vi "Periodic Tasks.vi"(8 "error in":errorcluster) -> ()   [LabVIEW 2017]
doc: "This VI runs in parallel to other tasks. It can contain as many user-defined periodic loops as you need. These can carry out PID or other sorts of timed response."
uses:
  <vilib>/Rock Robotics/WPI/ThirdParty/Phoenix-LabVIEW/Motor Controller/Controls/CTRE_Phoenix_MotorControl_FeedbackDevice.ctl
  <vilib>/Rock Robotics/WPI/ThirdParty/Phoenix-LabVIEW/Motor Controller/Controls/CTRE_Phoenix_MotorControl_StatusFrameEnhanced.ctl
  <vilib>/Rock Robotics/WPI/ThirdParty/Phoenix-LabVIEW/Motor Controller/Controls/CTRE_Phoenix_MotorControl_ControlMode.ctl
  <vilib>/Rock Robotics/WPI/ThirdParty/Phoenix-LabVIEW/Motor Controller/Controls/CTRE_Phoenix_MotorControl_TrajectoryPointTimeDur.ctl
  <vilib>/Rock Robotics/WPI/Utilities/WPI_GetSetVariantRefNum.vi
  <vilib>/Utility/file.llb/Read Delimited Spreadsheet (DBL).vi
panel:
  out "all rows 2":dbl[][](array[numeric])
  out "all rows":dbl[][](array[numeric])
  out "Mot Prof Active Velocity 2":dbl
  out "Mot Prof Active Position 2":dbl
  out "Mot Prof  Is Under Run 2":bool
  out "Mot Prof  Has Under Run 2":bool
  out "Mot Prof Active Is Last 2":bool
  out "Mot Prof Active Is Valid 2":bool
  out "Top Mot Prof Count 2":i32
  out "Btm Mot Prof Count 2":i32
  out "Btm Mot Prof Count":i32
  out "Sensor Out Of Phase":bool
  out "Loop Time":u32
  out "Points in the CSV":i32
  out "Mot Prof Active Position":dbl
  out "Mot Prof Active Velocity":dbl
  out "Top Mot Prof Count":i32
  out "Mot Prof Active Is Valid":bool
  out "Mot Prof Active Is Last":bool
  out "Mot Prof  Has Under Run":bool
  out "Mot Prof  Is Under Run":bool
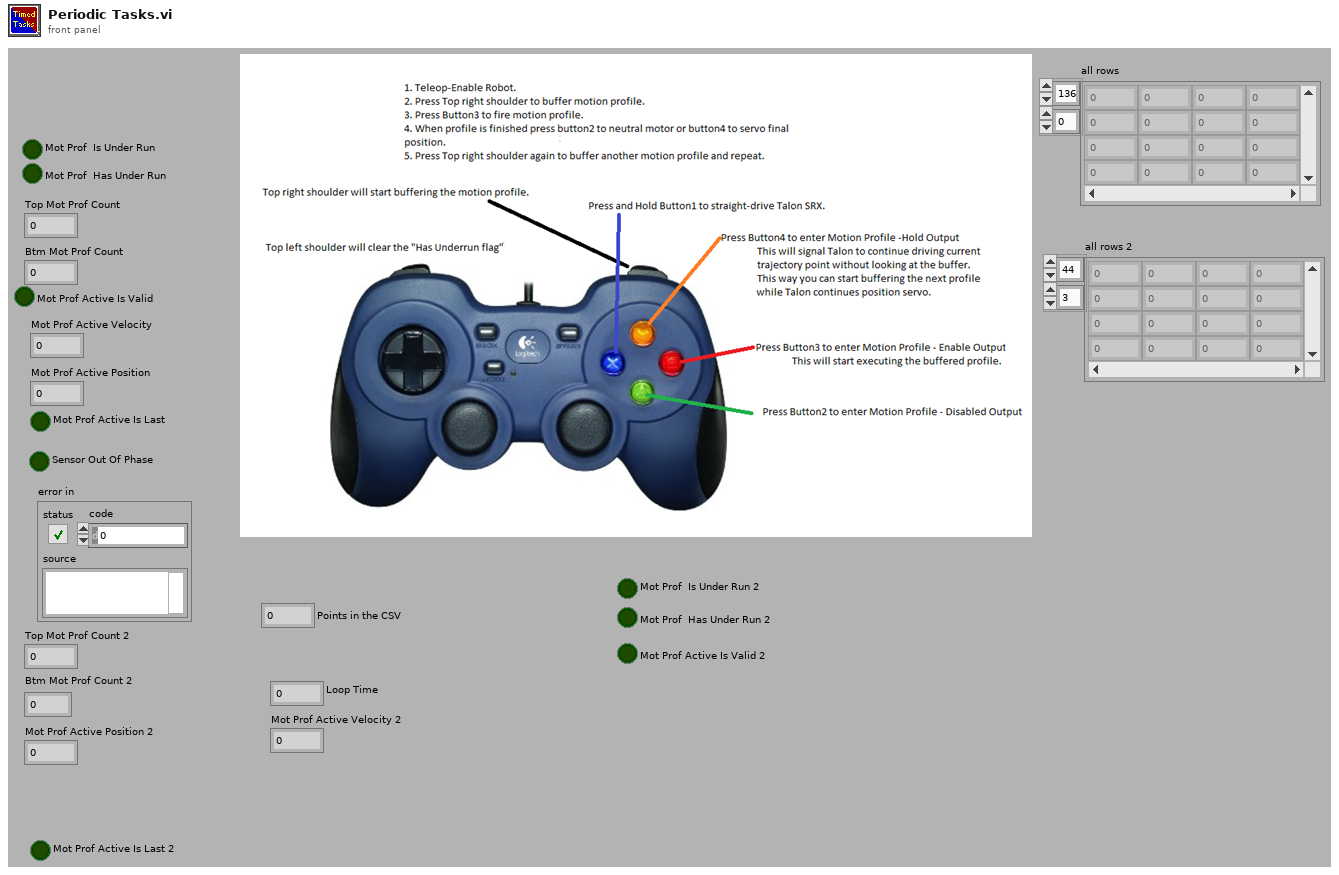
[diagram p1: front panel]
types:
  T1 = typedef "CTRE_Phoenix_MotorControl_StatusFrameEnhanced.ctl" = u16
  T2 = typedef "CTRE_Phoenix_MotorControl_FeedbackDevice.ctl" = i8
  T3 = typedef "WPI_MotorControlDeviceRef.ctl" = cluster{"DeviceStatus":errorcluster, "Type":T4, "PWM":cluster{"PWM Channel":T5, "DeadBand":T6}, "CAN":cluster{"Device Number":u8, "SetOutput VI Ref":variant, "GetOutput VI Ref":variant, "Enable VI Ref":variant, "Disable VI Ref":variant, "Data":variant}, "Invert":bool, "DIO PWM":cluster{"PWM \"Enable\" Channel":T5, "DIOChannel":T7, "PWM Rate":dbl}}
  T4 = typedef "WPI_MotorControlType.ctl" = enum16{"PWM", "CAN", "DIO PWM"}
  T5 = typedef "FPGA_DIOPWMChannel.ctl" = enum8{"PWM 0", "PWM 1", "PWM 2", "PWM 3", "PWM 4", "PWM 5", "PWM 6", "PWM 7", "PWM 8", "PWM 9", "PWM MXP 0", "PWM MXP 1", "PWM MXP 2", "PWM MXP 3", "PWM MXP 4", "PWM MXP 5", "PWM MXP 6", "PWM MXP 7", "PWM MXP 8", "PWM MXP 9", "Invalid"}
  T6 = typedef "WPI_PWMDeadband.ctl" = cluster{"Name":string, "maxPositivePwm":i32, "minPositivePwm":i32, "centerPwm":i32, "maxNegativePwm":i32, "minNegativePwm":i32, "angularRange":u16}
  T7 = typedef "FPGA_DIOChannel.ctl" = enum8{"DIO 0", "DIO 1", "DIO 2", "DIO 3", "DIO 4", "DIO 5", "DIO 6", "DIO 7", "DIO 8", "DIO 9", "DIO MXP 0", "DIO MXP 1", "DIO MXP 2", "DIO MXP 3", "DIO MXP 4", "DIO MXP 5", "DIO MXP 6", "DIO MXP 7", "DIO MXP 8", "DIO MXP 9", "DIO MXP 10", "DIO MXP 11", "DIO MXP 12", "DIO MXP 13", "DIO MXP 14", "DIO MXP 15", "SPI Port CS1", "SPI Port CS2", "SPI Port CS3", "SPI Port MISO", "SPI Port MOSI", "Invalid"}
  T8 = typedef "WPI_JoystickDevRef.ctl" = cluster{"Device":T9}
  T9 = typedef "WPI_JoystickDeviceEnum.ctl" = enum16{"USB 0", "USB 1", "USB 2", "USB 3", "USB 4", "USB 5"}
  T10 = typedef "CTRE_Phoenix_MotorControl_ControlMode.ctl" = u16
  T11 = cluster{"Under Voltage":bool, "Forward Limit Switch":bool, "Reverse Limit Switch":bool, "Forward Soft Limit":bool, "Reverse Soft Limit":bool, "Hardware Failure":bool, "Reset During Enable":bool, "Sensor Overflow":bool, "Sensor Out of Phase":bool, "Hardware ESD Reset":bool, "Remote Loss of Signal":bool}
  T12 = cluster{"Top Buffer Remaining":i32, "Top Buffer Count":i32, "Bottom Buffer Count":i32, "Has Underrun?":bool, "Is Underrun?":bool, "Active Point Valid?":bool, "Is Last?":bool, "Profile Slot Select 0":i32, "Output Enable":i32, "Time Duration (ms)":i32, "Profile Slot Select 1":i32}
  T13 = typedef "CTRE_Phoenix_MotorControl_TrajectoryPointTimeDur.ctl" = i32
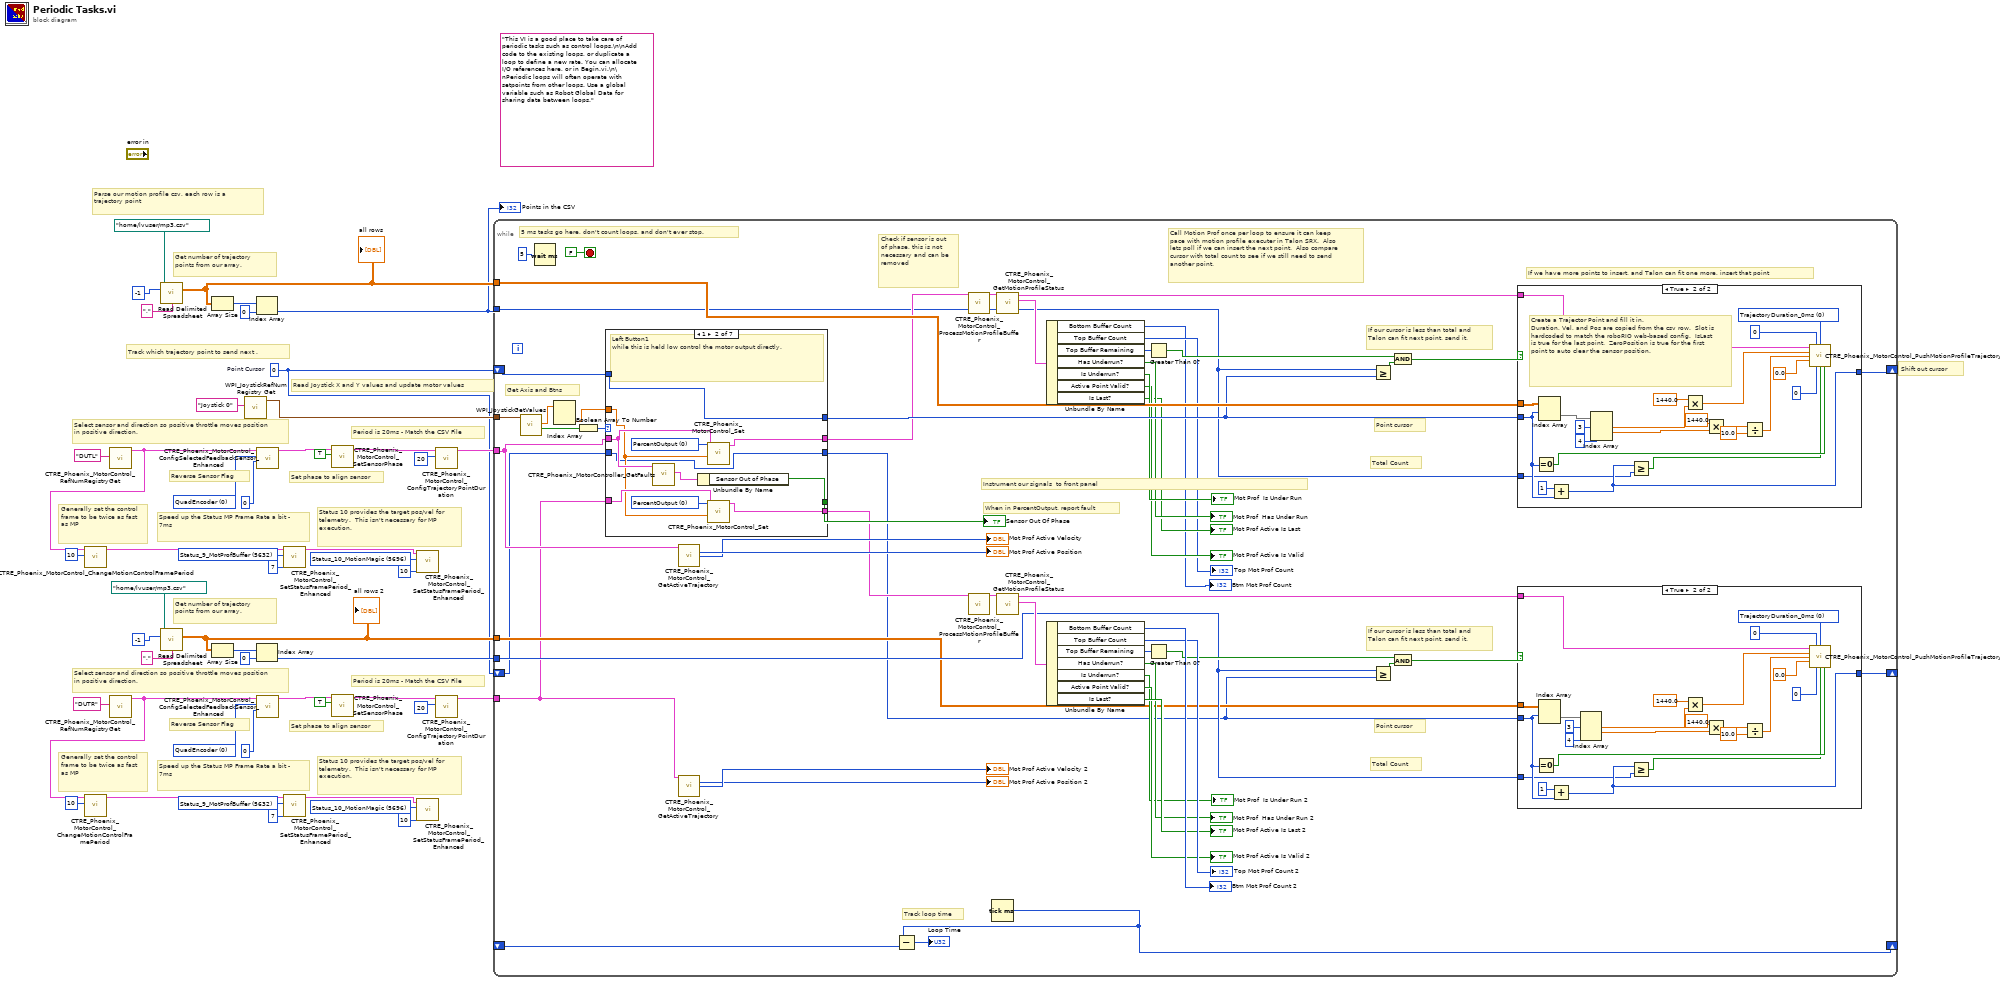
[diagram p0: block diagram]
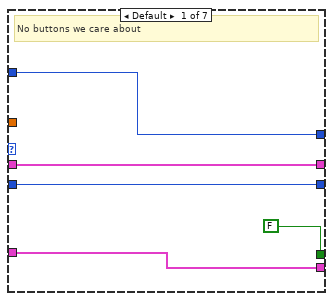
[diagram p3: hidden frame]
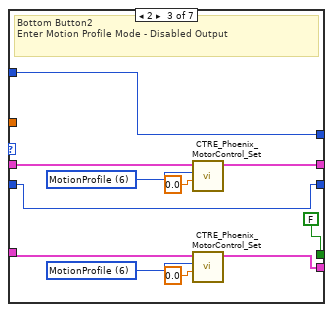
[diagram p4: hidden frame]
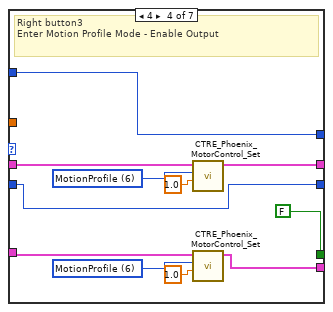
[diagram p5: hidden frame]
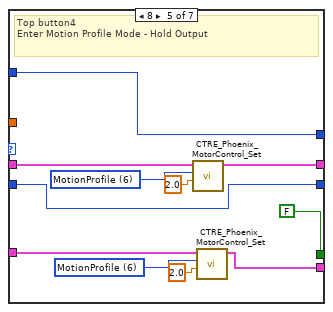
[diagram p6: hidden frame]
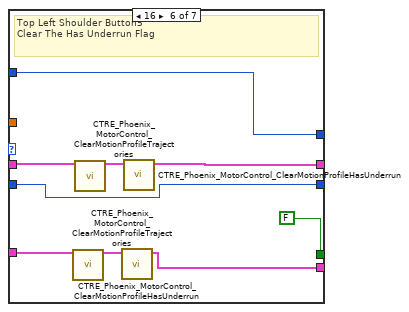
[diagram p7: hidden frame]
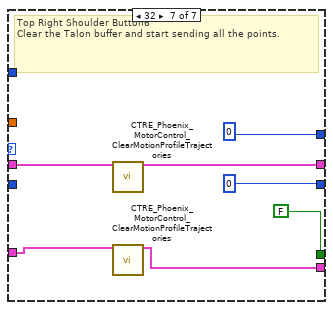
[diagram p8: hidden frame]
diagram:
  w18 = T1 5696 items=["Status_1_General"=5120, "Status_2_Feedback0"=5184, "Status_3_Quadrature"=5248, "Status_4_AinTempVbat"=5312, "Status_6_Misc"=5440, "Status_7_CommStatus"=5504, "Status_8_PulseWidth"=5568, "Status_9_MotProfBuffer"=5632, "Status_10_MotionMagic"=5696, "Status_11_UartGadgeteer"=5760, "Status_12_Feedback1"=5824, "Status_13_Base_PIDF0"=5888, "Status_14_Turn_PIDF1"=5952, "Status_15_FirmwareApiStatus"=6016] ("Status Frame")
  w14 = T1 5632 items=["Status_1_General"=5120, "Status_2_Feedback0"=5184, "Status_3_Quadrature"=5248, "Status_4_AinTempVbat"=5312, "Status_6_Misc"=5440, "Status_7_CommStatus"=5504, "Status_8_PulseWidth"=5568, "Status_9_MotProfBuffer"=5632, "Status_10_MotionMagic"=5696, "Status_11_UartGadgeteer"=5760, "Status_12_Feedback1"=5824, "Status_13_Base_PIDF0"=5888, "Status_14_Turn_PIDF1"=5952, "Status_15_FirmwareApiStatus"=6016] ("Status Frame")
  w12 = T2 0 items=["None"=-1, "QuadEncoder"=0, "Analog"=2, "Tachometer"=4, "Pulse Width Encoded Position"=8, "Sensor Sum (S0 + S1)"=9, "Sensor Difference (D0 - D1)"=10, "Remote Source 0"=11, "Remote Source 1"=12, "Software Emulated"=15] ("Feedback Device")
  w34 = T1 5696 items=["Status_1_General"=5120, "Status_2_Feedback0"=5184, "Status_3_Quadrature"=5248, "Status_4_AinTempVbat"=5312, "Status_6_Misc"=5440, "Status_7_CommStatus"=5504, "Status_8_PulseWidth"=5568, "Status_9_MotProfBuffer"=5632, "Status_10_MotionMagic"=5696, "Status_11_UartGadgeteer"=5760, "Status_12_Feedback1"=5824, "Status_13_Base_PIDF0"=5888, "Status_14_Turn_PIDF1"=5952, "Status_15_FirmwareApiStatus"=6016] ("Status Frame")
  w38 = T1 5632 items=["Status_1_General"=5120, "Status_2_Feedback0"=5184, "Status_3_Quadrature"=5248, "Status_4_AinTempVbat"=5312, "Status_6_Misc"=5440, "Status_7_CommStatus"=5504, "Status_8_PulseWidth"=5568, "Status_9_MotProfBuffer"=5632, "Status_10_MotionMagic"=5696, "Status_11_UartGadgeteer"=5760, "Status_12_Feedback1"=5824, "Status_13_Base_PIDF0"=5888, "Status_14_Turn_PIDF1"=5952, "Status_15_FirmwareApiStatus"=6016] ("Status Frame")
  w40 = T2 0 items=["None"=-1, "QuadEncoder"=0, "Analog"=2, "Tachometer"=4, "Pulse Width Encoded Position"=8, "Sensor Sum (S0 + S1)"=9, "Sensor Difference (D0 - D1)"=10, "Remote Source 0"=11, "Remote Source 1"=12, "Software Emulated"=15] ("Feedback Device")
  w3 = 0  # Point Cursor
  (unwired) "This VI is a good place to take care of periodic tasks such as control loops.\n\nAdd code to the existing loops, or duplicate a loop to define a new rate. You can allocate I/O references here, or in Begin.vi.\n\nPeriodic loops will often operate with setpoints from other loops. Use a global variable such as Robot Global Data for sharing data between loops."
  # "Get number of trajectory points from our array."
  # "Set phase to align sensor"
  # "Generally set the control frame to be twice as fast as MP"
  # "Status 10 provides the target pos/vel for telemetry.  This isn't necessary for MP execution."
  # "Period is 20ms - Match the CSV File"
  # "Reverse Sensor Flag"
  # "Select sensor and direction so positive throttle moves position in positive direction."
  # "Speed up the Status MP Frame Rate a bit - 7ms"
  # "Set phase to align sensor"
  # "Generally set the control frame to be twice as fast as MP"
  # "Status 10 provides the target pos/vel for telemetry.  This isn't necessary for MP execution."
  # "Period is 20ms - Match the CSV File"
  # "Shift out cursor"
  # "Read Joystick X and Y values and update motor values"
  # "Reverse Sensor Flag"
  # "Select sensor and direction so positive throttle moves position in positive direction."
  # "Get number of trajectory points from our array."
  # "Track which trajectory point to send next ."
  # "Speed up the Status MP Frame Rate a bit - 7ms"
  # "Parse our motion profile csv, each row is a trajectory point"
  n1 = call <vilib>:"CTRE_Phoenix_MotorControl_RefNumRegistryGet.vi"("refnum name"="DUTL") -> ("PhoenixMotorControlDevRef"=w29:T3)  [unwired: 9 in, 1 out]
  n2 = call <vilib>:"CTRE_Phoenix_MotorControl_ChangeMotionControlFramePeriod.vi"("periodMs"=10, "PhoenixMotorControlDevRef"=w29) -> ("PhoenixMotorControlDevRef"=w28:T3)  [unwired: 8 in, 1 out]
  n3 = call <vilib>:"CTRE_Phoenix_MotorControl_RefNumRegistryGet.vi"("refnum name"="DUTR") -> ("PhoenixMotorControlDevRef"=w22:T3)  [unwired: 9 in, 1 out]
  n4 = call <vilib>:"CTRE_Phoenix_MotorControl_ChangeMotionControlFramePeriod.vi"("periodMs"=10, "PhoenixMotorControlDevRef"=w22) -> ("PhoenixMotorControlDevRef"=w23:T3)  [unwired: 8 in, 1 out]
  n5 = call-poly <vilib>:"Read Delimited Spreadsheet.vi"("file path (dialog if empty)"=path "/home/lvuser/mp3.csv" ("file path (use dialog)"), "number of rows (all:-1)"=-1, "delimiter (\\t)"="," ("delimiter (\\t)")) -> ("all rows"=w42:dbl[][])  [unwired: 7 in, 5 out]
  "all rows" <- w42
  n6 = call-poly <vilib>:"Read Delimited Spreadsheet.vi"("file path (dialog if empty)"=path "/home/lvuser/mp3.csv" ("file path (use dialog)"), "number of rows (all:-1)"=-1, "delimiter (\\t)"="," ("delimiter (\\t)")) -> ("all rows"=w4:dbl[][])  [unwired: 7 in, 5 out]
  "all rows 2" <- w4
  n7 = Array Size(array=w42) -> (size(s)=w43:i32[])
  n8 = Array Size(array=w4) -> (size(s)=w9:i32[])
  n9 = call <vilib>:"WPI_JoystickRefNum Registry Get.vi"("refnum name"="Joystick 0") -> ("JoystickDevRef"=w47:T8)  [unwired: 1 in, 9 out]
  n10 = Index Array(array=w43, index=0) -> (element=w41:i32)
  "Points in the CSV" <- w41
  n11 = Index Array(array=w9, index=0) -> (element=w5:i32)
  n12 = call <vilib>:"CTRE_Phoenix_MotorControl_ConfigSelectedFeedbackSensor_Enhanced.vi"("pidLoopIdx"=0, "Feedback Device"=w40, "PhoenixMotorControlDevRef"=w29) -> ("PhoenixMotorControlDevRef"=w36:T3)  [unwired: 7 in, 1 out]
  n13 = call <vilib>:"CTRE_Phoenix_MotorControl_ConfigSelectedFeedbackSensor_Enhanced.vi"("pidLoopIdx"=0, "Feedback Device"=w12, "PhoenixMotorControlDevRef"=w22) -> ("PhoenixMotorControlDevRef"=w16:T3)  [unwired: 7 in, 1 out]
  n14 = call <vilib>:"CTRE_Phoenix_MotorControl_SetStatusFramePeriod_Enhanced.vi"("periodMs"=7, "Status Frame"=w38, "PhoenixMotorControlDevRef"=w28) -> ("PhoenixMotorControlDevRef"=w32:T3)  [unwired: 7 in, 1 out]
  n15 = call <vilib>:"CTRE_Phoenix_MotorControl_SetStatusFramePeriod_Enhanced.vi"("periodMs"=7, "Status Frame"=w14, "PhoenixMotorControlDevRef"=w23) -> ("PhoenixMotorControlDevRef"=w20:T3)  [unwired: 7 in, 1 out]
  n16 = call <vilib>:"CTRE_Phoenix_MotorControl_SetSensorPhase.vi"("PhaseSensor"=TRUE, "PhoenixMotorControlDevRef"=w36) -> ("PhoenixMotorControlDevRef"=w30:T3)  [unwired: 8 in, 1 out]
  n17 = call <vilib>:"CTRE_Phoenix_MotorControl_SetSensorPhase.vi"("PhaseSensor"=TRUE, "PhoenixMotorControlDevRef"=w16) -> ("PhoenixMotorControlDevRef"=w21:T3)  [unwired: 8 in, 1 out]
  n18 = call <vilib>:"CTRE_Phoenix_MotorControl_SetStatusFramePeriod_Enhanced.vi"("periodMs"=10, "Status Frame"=w34, "PhoenixMotorControlDevRef"=w32) -> ()  [unwired: 7 in, 2 out]
  n19 = call <vilib>:"CTRE_Phoenix_MotorControl_SetStatusFramePeriod_Enhanced.vi"("periodMs"=10, "Status Frame"=w18, "PhoenixMotorControlDevRef"=w20) -> ()  [unwired: 7 in, 2 out]
  n20 = call <vilib>:"CTRE_Phoenix_MotorControl_ConfigTrajectoryPointDuration.vi"("durationMs"=20 ("periodMs"), "PhoenixMotorControlDevRef"=w30) -> ("PhoenixMotorControlDevRef"=w31:T3)  [unwired: 8 in, 1 out]
  n21 = call <vilib>:"CTRE_Phoenix_MotorControl_ConfigTrajectoryPointDuration.vi"("durationMs"=20 ("periodMs"), "PhoenixMotorControlDevRef"=w21) -> ("PhoenixMotorControlDevRef"=w10:T3)  [unwired: 8 in, 1 out]
  n22 = while {
    tunnel: w47 -> [w102]
    tunnel: w42 -> [w101]
    shift-right: [w100] -> _
    shift-left: w3 -> [w99]
    tunnel: w41 -> [w72]
    tunnel: w31 -> [w76]
    shift-right: [w79] -> _
    shift-left: _ -> [w78]
    tunnel: w10 -> [w50]
    tunnel: w5 -> [w57]
    tunnel: w4 -> [w56]
    shift-right: [w55] -> _
    shift-left: w3 -> [w53]
    stop <- FALSE stop-if-true
    # "Point cursor"
    # "Total Count"
    # "If our cursor is less than total and Talon can fit next point, send it."
    # "Track loop time"
    # "When in PercentOutput, report fault"
    # "Check if sensor is out of phase, this is not necessary and can be removed"
    # "Call Motion Prof once per loop to ensure it can keep pace with motion profile executer in Talon SRX.  Also lets poll if we can insert the next point.  Also compare cursor with total count to see if we still need to send another point."
    # "Instrument our signals  to front panel"
    # "Get Axis and Btns"
    # "Point cursor"
    # "Total Count"
    # "If our cursor is less than total and Talon can fit next point, send it."
    # "If we have more points to insert, and Talon can fit one more, insert that point"
    # "5 ms tasks go here, don't count loops, and don't ever stop."
    n23 = call <vilib>:"WPI_JoystickGetValues.vi"("JoystickDevRef"=w102) -> ("Buttons"=w92:bool[], "Axes"=w93:dbl[])  [unwired: 6 in, 3 out]
    n24 = Wait (ms)(milliseconds to wait=u32 5) -> ()  [unwired: 1 out]
    n25 = Index Array(array=w93) -> (element #2=w90:dbl)  [unwired: 2 in, 1 out]
    n26 = Boolean Array To Number(Boolean array=w92) -> (number=w91:u32)
    n27 = case shown="1" w91 {
      tunnel: w76 -> [w133 w142 w153 w164 w177 w184 w191]
      tunnel: [w133 w140 w152 w163 w174 w185 w192] -> w74
      tunnel: w90 -> [_ w135 _ _ _ _ _]
      tunnel: [w132 w144 w151 w162 w173 w186 0 ("Capacity")] -> w97
      tunnel: w99 -> [w132 w144 w151 w162 w173 w186 _]
      tunnel: [FALSE ("Sensor Out of Phase") w139 FALSE ("Sensor Out of Phase") FALSE ("Sensor Out of Phase") FALSE ("Sensor Out of Phase") FALSE ("Sensor Out of Phase") FALSE ("Sensor Out of Phase")] -> w73
      tunnel: [w130 w137 w146 w157 w168 w180 w187] -> w58
      tunnel: w50 -> [w130 w136 w147 w158 w169 w179 w188]
      tunnel: [w129 w134 w145 w156 w167 w178 0 ("Capacity")] -> w54
      tunnel: w53 -> [w129 w134 w145 w156 w167 w178 _]
      frame Default {
        # "No buttons we care about"
      }
      frame 1 {
        w138 = T10 0 items=["PercentOutput"=0, "Position"=1, "Velocity"=2, "Current"=3, "Follower"=5, "MotionProfile"=6, "MotionMagic"=7, "MotionMagicArc"=8, "MotionProfileArc"=10, "Disabled"=15] ("Control Mode")
        w143 = T10 0 items=["PercentOutput"=0, "Position"=1, "Velocity"=2, "Current"=3, "Follower"=5, "MotionProfile"=6, "MotionMagic"=7, "MotionMagicArc"=8, "MotionProfileArc"=10, "Disabled"=15] ("Control Mode")
        # "Left Button1\nwhile this is held low control the motor output directly."
        n28 = call <vilib>:"CTRE_Phoenix_MotorController_GetFaults.vi"("PhoenixMotorControlDevRef"=w142) -> ("Faults"=w141:T11)  [unwired: 8 in, 2 out]
        n29 = Unbundle By Name(w141) -> ("Sensor Out of Phase"=w139:bool)
        n30 = call <vilib>:"CTRE_Phoenix_MotorControl_Set.vi"("Output"=w135, "Control Mode"=w143, "PhoenixMotorControlDevRef"=w142) -> ("PhoenixMotorControlDevRef"=w140:T3)  [unwired: 7 in, 1 out]
        n31 = call <vilib>:"CTRE_Phoenix_MotorControl_Set.vi"("Output"=w135, "Control Mode"=w138, "PhoenixMotorControlDevRef"=w136) -> ("PhoenixMotorControlDevRef"=w137:T3)  [unwired: 7 in, 1 out]
      }
      frame 2 {
        w148 = T10 6 items=["PercentOutput"=0, "Position"=1, "Velocity"=2, "Current"=3, "Follower"=5, "MotionProfile"=6, "MotionMagic"=7, "MotionMagicArc"=8, "MotionProfileArc"=10, "Disabled"=15] ("Control Mode")
        w155 = T10 6 items=["PercentOutput"=0, "Position"=1, "Velocity"=2, "Current"=3, "Follower"=5, "MotionProfile"=6, "MotionMagic"=7, "MotionMagicArc"=8, "MotionProfileArc"=10, "Disabled"=15] ("Control Mode")
        # "Bottom Button2\nEnter Motion Profile Mode - Disabled Output"
        n32 = call <vilib>:"CTRE_Phoenix_MotorControl_Set.vi"("Output"=0.0, "Control Mode"=w155, "PhoenixMotorControlDevRef"=w153) -> ("PhoenixMotorControlDevRef"=w152:T3)  [unwired: 7 in, 1 out]
        n33 = call <vilib>:"CTRE_Phoenix_MotorControl_Set.vi"("Output"=0.0, "Control Mode"=w148, "PhoenixMotorControlDevRef"=w147) -> ("PhoenixMotorControlDevRef"=w146:T3)  [unwired: 7 in, 1 out]
      }
      frame 4 {
        w159 = T10 6 items=["PercentOutput"=0, "Position"=1, "Velocity"=2, "Current"=3, "Follower"=5, "MotionProfile"=6, "MotionMagic"=7, "MotionMagicArc"=8, "MotionProfileArc"=10, "Disabled"=15] ("Control Mode")
        w166 = T10 6 items=["PercentOutput"=0, "Position"=1, "Velocity"=2, "Current"=3, "Follower"=5, "MotionProfile"=6, "MotionMagic"=7, "MotionMagicArc"=8, "MotionProfileArc"=10, "Disabled"=15] ("Control Mode")
        # "Right button3\nEnter Motion Profile Mode - Enable Output"
        n34 = call <vilib>:"CTRE_Phoenix_MotorControl_Set.vi"("Output"=1.0, "Control Mode"=w166, "PhoenixMotorControlDevRef"=w164) -> ("PhoenixMotorControlDevRef"=w163:T3)  [unwired: 7 in, 1 out]
        n35 = call <vilib>:"CTRE_Phoenix_MotorControl_Set.vi"("Output"=1.0, "Control Mode"=w159, "PhoenixMotorControlDevRef"=w158) -> ("PhoenixMotorControlDevRef"=w157:T3)  [unwired: 7 in, 1 out]
      }
      frame 8 {
        w170 = T10 6 items=["PercentOutput"=0, "Position"=1, "Velocity"=2, "Current"=3, "Follower"=5, "MotionProfile"=6, "MotionMagic"=7, "MotionMagicArc"=8, "MotionProfileArc"=10, "Disabled"=15] ("Control Mode")
        w176 = T10 6 items=["PercentOutput"=0, "Position"=1, "Velocity"=2, "Current"=3, "Follower"=5, "MotionProfile"=6, "MotionMagic"=7, "MotionMagicArc"=8, "MotionProfileArc"=10, "Disabled"=15] ("Control Mode")
        # "Top button4\nEnter Motion Profile Mode - Hold Output"
        n36 = call <vilib>:"CTRE_Phoenix_MotorControl_Set.vi"("Output"=2.0, "Control Mode"=w176, "PhoenixMotorControlDevRef"=w177) -> ("PhoenixMotorControlDevRef"=w174:T3)  [unwired: 7 in, 1 out]
        n37 = call <vilib>:"CTRE_Phoenix_MotorControl_Set.vi"("Output"=2.0, "Control Mode"=w170, "PhoenixMotorControlDevRef"=w169) -> ("PhoenixMotorControlDevRef"=w168:T3)  [unwired: 7 in, 1 out]
      }
      frame 16 {
        # "Top Left Shoulder Button5\nClear The Has Underrun Flag"
        n38 = call <vilib>:"CTRE_Phoenix_MotorControl_ClearMotionProfileTrajectories.vi"("PhoenixMotorControlDevRef"=w179) -> ("PhoenixMotorControlDevRef"=w181:T3)  [unwired: 13 in, 1 out]
        n39 = call <vilib>:"CTRE_Phoenix_MotorControl_ClearMotionProfileTrajectories.vi"("PhoenixMotorControlDevRef"=w184) -> ("PhoenixMotorControlDevRef"=w183:T3)  [unwired: 13 in, 1 out]
        n40 = call <vilib>:"CTRE_Phoenix_MotorControl_ClearMotionProfileHasUnderrun.vi"("PhoenixMotorControlDevRef"=w181) -> ("PhoenixMotorControlDevRef"=w180:T3)  [unwired: 9 in, 1 out]
        n41 = call <vilib>:"CTRE_Phoenix_MotorControl_ClearMotionProfileHasUnderrun.vi"("PhoenixMotorControlDevRef"=w183) -> ("PhoenixMotorControlDevRef"=w185:T3)  [unwired: 9 in, 1 out]
      }
      frame 32 {
        # "Top Right Shoulder Button6\nClear the Talon buffer and start sending all the points."
        n42 = call <vilib>:"CTRE_Phoenix_MotorControl_ClearMotionProfileTrajectories.vi"("PhoenixMotorControlDevRef"=w191) -> ("PhoenixMotorControlDevRef"=w192:T3)  [unwired: 13 in, 1 out]
        n43 = call <vilib>:"CTRE_Phoenix_MotorControl_ClearMotionProfileTrajectories.vi"("PhoenixMotorControlDevRef"=w188) -> ("PhoenixMotorControlDevRef"=w187:T3)  [unwired: 13 in, 1 out]
      }
    }
    "Sensor Out Of Phase" <- w73
    n44 = call <vilib>:"CTRE_Phoenix_MotorControl_GetActiveTrajectory.vi"("PhoenixMotorControlDevRef"=w76) -> ("Position (Sensor Units)"=→"Mot Prof Active Position":i32, "Velocity (Sensor Units per 100 ms)"=→"Mot Prof Active Velocity":i32)  [unwired: 10 in, 3 out]
    n45 = call <vilib>:"CTRE_Phoenix_MotorControl_GetActiveTrajectory.vi"("PhoenixMotorControlDevRef"=w50) -> ("Position (Sensor Units)"=→"Mot Prof Active Position 2":i32, "Velocity (Sensor Units per 100 ms)"=→"Mot Prof Active Velocity 2":i32)  [unwired: 10 in, 3 out]
    n46 = call <vilib>:"CTRE_Phoenix_MotorControl_ProcessMotionProfileBuffer.vi"("PhoenixMotorControlDevRef"=w74) -> ("PhoenixMotorControlDevRef"=w87:T3)  [unwired: 13 in, 1 out]
    n47 = call <vilib>:"CTRE_Phoenix_MotorControl_ProcessMotionProfileBuffer.vi"("PhoenixMotorControlDevRef"=w58) -> ("PhoenixMotorControlDevRef"=w65:T3)  [unwired: 13 in, 1 out]
    n48 = Tick Count (ms)() -> (millisecond timer value=w79:u32)
    n49 = Subtract(x=w79, y=w78) -> (x-y=→"Loop Time":u32)
    n50 = call <vilib>:"CTRE_Phoenix_MotorControl_GetMotionProfileStatus.vi"("PhoenixMotorControlDevRef"=w87) -> ("Motion Profile Status"=w89:T12, "PhoenixMotorControlDevRef"=w95:T3)  [unwired: 8 in, 1 out]
    n51 = call <vilib>:"CTRE_Phoenix_MotorControl_GetMotionProfileStatus.vi"("PhoenixMotorControlDevRef"=w65) -> ("Motion Profile Status"=w63:T12, "PhoenixMotorControlDevRef"=w61:T3)  [unwired: 8 in, 1 out]
    n52 = Unbundle By Name(w89) -> ("Bottom Buffer Count"=→"Btm Mot Prof Count":i32, "Top Buffer Count"=→"Top Mot Prof Count":i32, "Top Buffer Remaining"=w88:i32, "Has Underrun?"=→"Mot Prof  Has Under Run":bool, "Is Underrun?"=→"Mot Prof  Is Under Run":bool, "Active Point Valid?"=→"Mot Prof Active Is Valid":bool, "Is Last?"=→"Mot Prof Active Is Last":bool)
    n53 = Unbundle By Name(w63) -> ("Bottom Buffer Count"=→"Btm Mot Prof Count 2":i32, "Top Buffer Count"=→"Top Mot Prof Count 2":i32, "Top Buffer Remaining"=w64:i32, "Has Underrun?"=→"Mot Prof  Has Under Run 2":bool, "Is Underrun?"=→"Mot Prof  Is Under Run 2":bool, "Active Point Valid?"=→"Mot Prof Active Is Valid 2":bool, "Is Last?"=→"Mot Prof Active Is Last 2":bool)
    n54 = Greater Than 0?(x=w88) -> (x > 0?=w94:bool)
    n55 = Greater Than 0?(x=w64) -> (x > 0?=w62:bool)
    n56 = Greater Or Equal?(x=w72, y=w97) -> (x >= y?=w96:bool)
    n57 = Greater Or Equal?(x=w57, y=w54) -> (x >= y?=w60:bool)
    n58 = And(x=w94, y=w96) -> (x .and. y?=w98:bool)
    n59 = And(x=w62, y=w60) -> (x .and. y?=w59:bool)
    n60 = case shown="True" w98 {
      tunnel: w101 -> [_ w217]
      tunnel: [w194 w213] -> w100
      tunnel: w97 -> [w194 w214]
      tunnel: w72 -> [_ w212]
      tunnel: w95 -> [_ w211]
      frame False {
      }
      frame True {
        w198 = T13 0 items=["TrajectoryDuration_0ms"=0, "TrajectoryDuration_5ms"=5, "TrajectoryDuration_10ms"=10, "TrajectoryDuration_20ms"=20, "TrajectoryDuration_30ms"=30, "TrajectoryDuration_40ms"=40, "TrajectoryDuration_50ms"=50, "TrajectoryDuration_100ms"=100] ("durationMs")
        # "Create a Trajector Point and fill it in.\nDuration, Vel, and Pos are copied from the csv row.  Slot is hardcoded to match the roboRIO web-based config.  IsLast is true for the last point.  ZeroPosition is true for the first point to auto clear the sensor position."
        n61 = Equal To 0?(x=w214) -> (x = 0?=w209:bool)
        n62 = Index Array(array=w217, index (row)=w214) -> (element=w215:dbl[])  [unwired: 1 in]
        n63 = Add(x=u32 1, y=w214) -> (x+y=w213:u32)
        n64 = Index Array(array=w215, index #1=3 ("index"), index #2=4 ("index")) -> (element #1=w205:dbl, element #2=w202:dbl)  [unwired: 1 in, 1 out]
        n65 = Greater Or Equal?(x=w213, y=w212) -> (x >= y?=w208:bool)
        n66 = Multiply(x=1440.0, y=w205) -> (x*y=w204:dbl)
        n67 = Multiply(x=1440.0, y=w202) -> (x*y=w200:dbl)
        n68 = Divide(x=w200, y=10.0) -> (x/y=w199:dbl)
        n69 = call <vilib>:"CTRE_Phoenix_MotorControl_PushMotionProfileTrajectory.vi"("PhoenixMotorControlDevRef"=w211, "profileSlotSelect1"=0, "durationMs"=w198, "position"=w204, "velocity"=w199, "auxiliaryPos"=0.0 ("headingDeg"), "profileSlotSelect0"=0, "isLastPoint?"=w208, "Zero Position?"=w209) -> ()  [unwired: 5 in, 2 out]
      }
    }
    n70 = case shown="True" w59 {
      tunnel: w56 -> [_ w128]
      tunnel: [w105 w124] -> w55
      tunnel: w54 -> [w105 w125]
      tunnel: w57 -> [_ w123]
      tunnel: w61 -> [_ w122]
      frame False {
      }
      frame True {
        w109 = T13 0 items=["TrajectoryDuration_0ms"=0, "TrajectoryDuration_5ms"=5, "TrajectoryDuration_10ms"=10, "TrajectoryDuration_20ms"=20, "TrajectoryDuration_30ms"=30, "TrajectoryDuration_40ms"=40, "TrajectoryDuration_50ms"=50, "TrajectoryDuration_100ms"=100] ("durationMs")
        n71 = Equal To 0?(x=w125) -> (x = 0?=w120:bool)
        n72 = Index Array(array=w128, index (row)=w125) -> (element=w126:dbl[])  [unwired: 1 in]
        n73 = Add(x=u32 1, y=w125) -> (x+y=w124:u32)
        n74 = Index Array(array=w126, index #1=3 ("index"), index #2=4 ("index")) -> (element #1=w116:dbl, element #2=w113:dbl)  [unwired: 1 in, 1 out]
        n75 = Greater Or Equal?(x=w124, y=w123) -> (x >= y?=w119:bool)
        n76 = Multiply(x=1440.0, y=w116) -> (x*y=w115:dbl)
        n77 = Multiply(x=1440.0, y=w113) -> (x*y=w111:dbl)
        n78 = Divide(x=w111, y=10.0) -> (x/y=w110:dbl)
        n79 = call <vilib>:"CTRE_Phoenix_MotorControl_PushMotionProfileTrajectory.vi"("PhoenixMotorControlDevRef"=w122, "profileSlotSelect1"=0, "durationMs"=w109, "position"=w115, "velocity"=w110, "auxiliaryPos"=0.0 ("headingDeg"), "profileSlotSelect0"=0, "isLastPoint?"=w119, "Zero Position?"=w120) -> ()  [unwired: 5 in, 2 out]
      }
    }
  }
